vi "dfd_Expand PZ Orders.vi"(2 "zeros":T1[](array[typedef]), 3 "poles":T1[](array[typedef])) -> (0 "zeros expanded":T1[](array[typedef]), 1 "poles expanded":T1[](array[typedef]))   [LabVIEW 2017, in "NI_DigFilter_Design.lvlib"]
uses:
  <vilib>/addons/Digital Filter Design/NI_DigFilter_Design.lvlib
  <vilib>/addons/Digital Filter Design/_Objects.llb/DFD Pole-Zero.ctl
  <vilib>/addons/Digital Filter Design/NI_DigFilterLicensed.lvlib
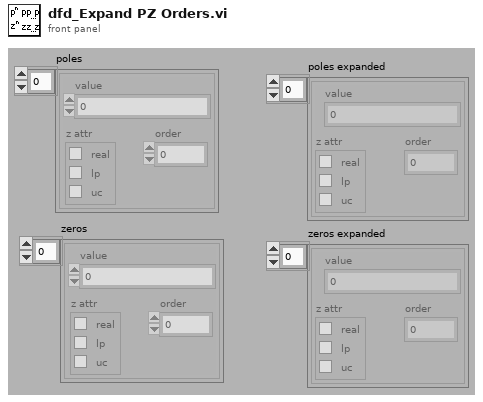
[diagram p1: front panel]
types:
  T1 = typedef "NI_DigFilterLicensed.lvlib/DFD Pole-Zero.ctl" = cluster{"value":cdb, "z attr":cluster{"real":bool, "lp":bool, "uc":bool}, "order":i32}
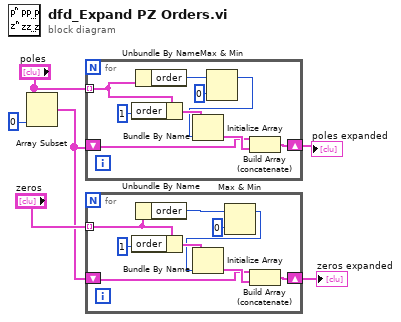
[diagram p0: block diagram]
diagram:
  n1 = Array Subset(array="poles", length=0) -> (w2:T1[])  [unwired: 1 in]
  n2 = for {
    shift-right: [w11] -> w4
    shift-left: w2 -> [w10]
    tunnel: "poles" -> [w14] mode=indexing
    n3 = Bundle By Name(cluster=w14, "order"=1) -> (w13:T1)
    n4 = Unbundle By Name(w14) -> ("order"=w8:i32)
    n5 = Max & Min(x=w8, y=0) -> (max(x,y)=w7:i32)  [unwired: 1 out]
    n6 = Initialize Array(w13, w7) -> (w12:T1[])
    n7 = Build Array (concatenate)(w10, w12) -> (w11:T1[])
  }
  "poles expanded" <- w4
  n8 = for {
    shift-right: [w21] -> w1
    shift-left: w2 -> [w20]
    tunnel: "zeros" -> [w19] mode=indexing
    n9 = Bundle By Name(cluster=w19, "order"=1) -> (w23:T1)
    n10 = Unbundle By Name(w19) -> ("order"=w17:i32)
    n11 = Max & Min(x=w17, y=0) -> (max(x,y)=w16:i32)  [unwired: 1 out]
    n12 = Initialize Array(w23, w16) -> (w22:T1[])
    n13 = Build Array (concatenate)(w20, w22) -> (w21:T1[])
  }
  "zeros expanded" <- w1
